vi "ZCAN_Send_Multiframe.vi"(4 "CAN_CH":u8, 5 "CANFD_SpeedUp":u32, 6 "SendData":string="11 22 33 44 55 66 77 88", 7 "ID":u32=18 format="0x%08x", 8 "error in":errorcluster, 9 "agreement":T1, 10 "frame type":T2, 11 "can_index_handle":u32) -> (0 "error out":errorcluster, 3 "Send,DataOut":string)   [LabVIEW 2020]
uses:
  data_type/frame type.ctl
  data_type/Agreement.ctl
  data_type/ZCAN_TransmitFD_frame.ctl
  c76635de-1d19-4bb1-8ca9-fd1db6ddedf1.vi
  zlgcan.lvlib
panel:
  in  "Wait_ms":i32
  in  "Send FillUp":string="AA"
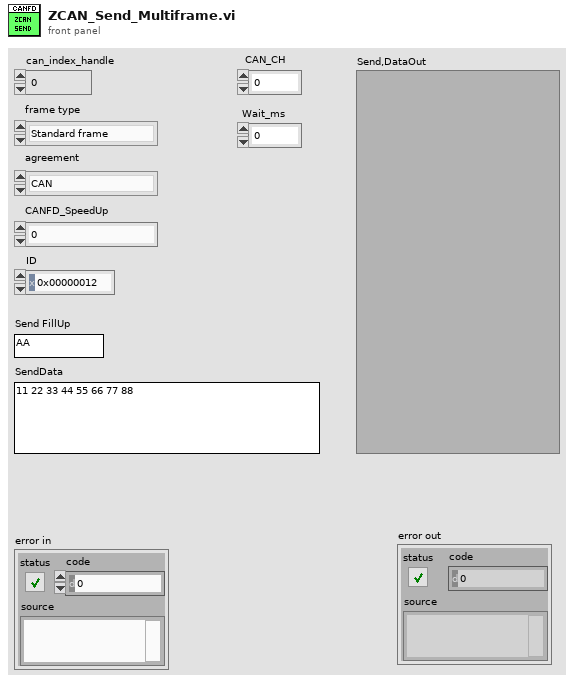
[diagram p1: front panel]
types:
  T1 = typedef "zlgcan.lvlib/Agreement.ctl" = enum16{"CAN", "CANFD"}
  T2 = typedef "zlgcan.lvlib/frame type.ctl" = enum32{"Standard frame", "Extended frame"}
  T3 = typedef "zlgcan.lvlib/ZCAN_TransmitFD_frame.ctl" = cluster{"帧类型":u32, "帧格式":u32, "ID":u32, "数据长度":u8, "CANFD加速？":u8, "DATA":cluster{"CAN数据[0]":u8, "CAN数据[1]":u8, "CAN数据[2]":u8, "CAN数据[3]":u8, "CAN数据[4]":u8, "CAN数据[5]":u8, "CAN数据[6]":u8, "CAN数据[7]":u8, "CAN数据[8]":u8, "CAN数据[9]":u8, "CAN数据[10]":u8, "CAN数据[11] ":u8, "CAN数据[12] ":u8, "CAN数据[13] ":u8, "CAN数据[14] ":u8, "CAN数据[15] ":u8, "CAN数据[16]":u8, "CAN数据[17]":u8, "CAN数据[18]":u8, "CAN数据[19]":u8, "CAN数据[20]":u8, "CAN数据[21]":u8, "CAN数据[22]":u8, "CAN数据[23]":u8, "CAN数据[24] ":u8, "CAN数据[25]":u8, "CAN数据[26]":u8, "CAN数据[27]":u8, "CAN数据[28]":u8, "CAN数据[29]":u8, "CAN数据[30]":u8, "CAN数据[31]":u8, "CAN数据[32]":u8, "CAN数据[33]":u8, "CAN数据[34]":u8, "CAN数据[35]":u8, "CAN数据[36]":u8, "CAN数据[37]":u8, "CAN数据[38]":u8, "CAN数据[39]":u8, "CAN数据[40]":u8, "CAN数据[41]":u8, "CAN数据[42]":u8, "CAN数据[43]":u8, "CAN数据[44]":u8, "CAN数据[45]":u8, "CAN数据[46]":u8, "CAN数据[47]":u8, "CAN数据[48]":u8, "CAN数据[49]":u8, "CAN数据[50]":u8, "CAN数据[51]":u8, "CAN数据[52]":u8, "CAN数据[53]":u8, "CAN数据[54]":u8, "CAN数据[55]":u8, "CAN数据[56]":u8, "CAN数据[57]":u8, "CAN数据[58]":u8, "CAN数据[59]":u8, "CAN数据[60]":u8, "CAN数据[61]":u8, "CAN数据[62]":u8, "CAN数据[63]":u8}}
  T4 = cluster{"u8 Data[][0]":u8, "u8 Data[][1]":u8, "u8 Data[][2]":u8, "u8 Data[][3]":u8, "u8 Data[][4]":u8, "u8 Data[][5]":u8, "u8 Data[][6]":u8, "u8 Data[][7]":u8, "u8 Data[][8]":u8, "u8 Data[][9]":u8, "u8 Data[][10]":u8, "u8 Data[][11]":u8, "u8 Data[][12]":u8, "u8 Data[][13]":u8, "u8 Data[][14]":u8, "u8 Data[][15]":u8, "u8 Data[][16]":u8, "u8 Data[][17]":u8, "u8 Data[][18]":u8, "u8 Data[][19]":u8, "u8 Data[][20]":u8, "u8 Data[][21]":u8, "u8 Data[][22]":u8, "u8 Data[][23]":u8, "u8 Data[][24]":u8, "u8 Data[][25]":u8, "u8 Data[][26]":u8, "u8 Data[][27]":u8, "u8 Data[][28]":u8, "u8 Data[][29]":u8, "u8 Data[][30]":u8, "u8 Data[][31]":u8, "u8 Data[][32]":u8, "u8 Data[][33]":u8, "u8 Data[][34]":u8, "u8 Data[][35]":u8, "u8 Data[][36]":u8, "u8 Data[][37]":u8, "u8 Data[][38]":u8, "u8 Data[][39]":u8, "u8 Data[][40]":u8, "u8 Data[][41]":u8, "u8 Data[][42]":u8, "u8 Data[][43]":u8, "u8 Data[][44]":u8, "u8 Data[][45]":u8, "u8 Data[][46]":u8, "u8 Data[][47]":u8, "u8 Data[][48]":u8, "u8 Data[][49]":u8, "u8 Data[][50]":u8, "u8 Data[][51]":u8, "u8 Data[][52]":u8, "u8 Data[][53]":u8, "u8 Data[][54]":u8, "u8 Data[][55]":u8, "u8 Data[][56]":u8, "u8 Data[][57]":u8, "u8 Data[][58]":u8, "u8 Data[][59]":u8, "u8 Data[][60]":u8, "u8 Data[][61]":u8, "u8 Data[][62]":u8, "u8 Data[][63]":u8}
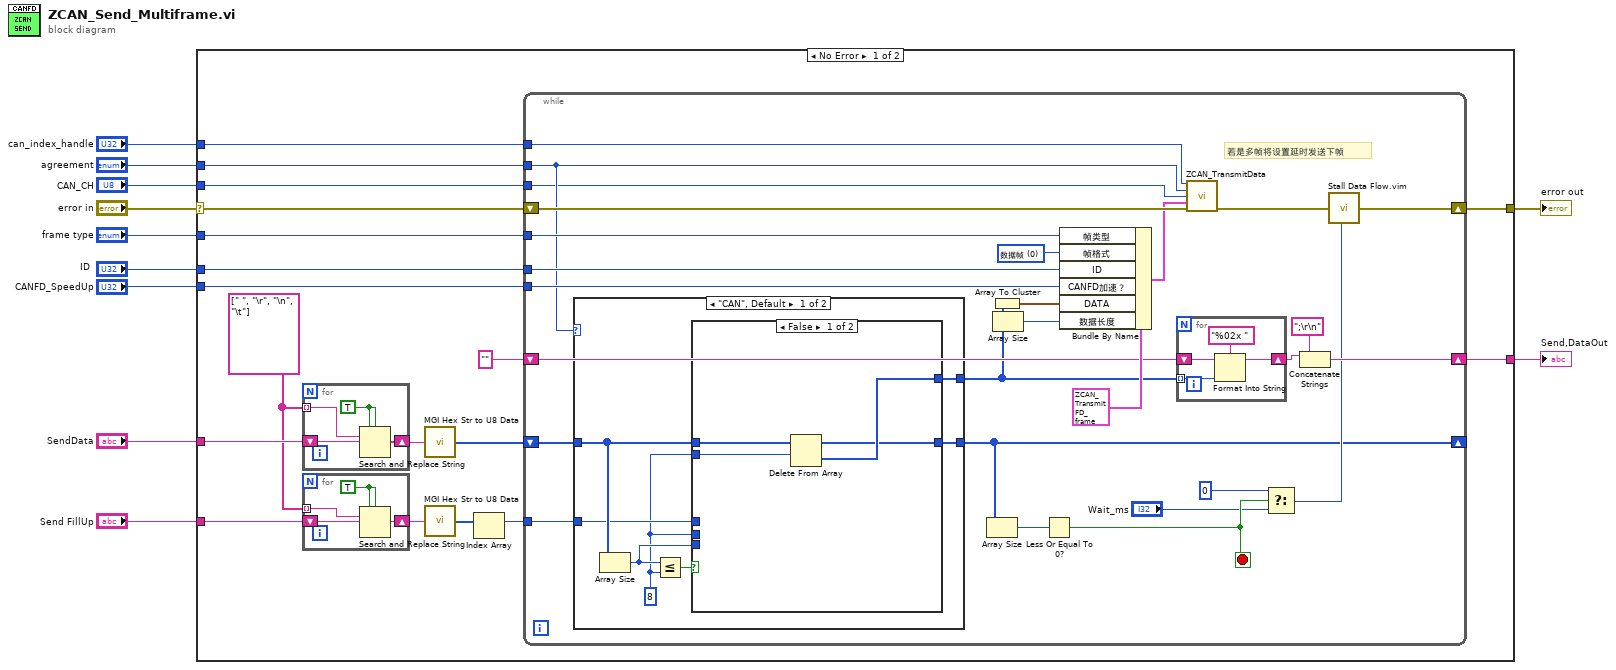
[diagram p0: block diagram]
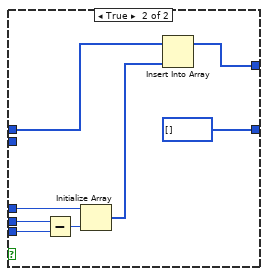
[diagram p2: hidden frame]
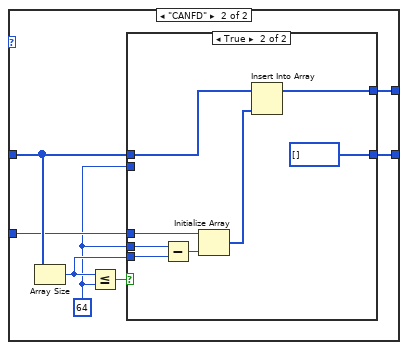
[diagram p3: hidden frame]
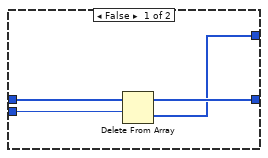
[diagram p4: hidden frame]
diagram:
  n1 = case shown="No Error" "error in" {
    selector: "error in" -> [w29 w108]
    tunnel: [w28 w108] -> w10
    tunnel: "can_index_handle" -> [w27 _]
    tunnel: "frame type" -> [w26 _]
    tunnel: "ID" -> [w25 _]
    tunnel: "CANFD_SpeedUp" -> [w24 _]
    tunnel: "SendData" -> [w22 w107]
    tunnel: "agreement" -> [w18 _]
    tunnel: [w16 w107] -> w3
    tunnel: "CAN_CH" -> [w15 _]
    tunnel: "Send FillUp" -> [w13 _]
    frame No Error {
      w12 = string[] [" ", "\r", "\n", "\t"] ("search string")
      n2 = for {
        tunnel: w12 -> [w35] mode=indexing
        shift-right: [w37] -> w23
        shift-left: w22 -> [w36]
        w34 = TRUE ("replace all? (F)")
        n3 = Search and Replace String(replace all?=w34, case sensitive?=w34, input string=w36, search string=w35) -> (result string=w37:string)  [unwired: 4 in, 3 out]
      }
      n4 = for {
        tunnel: w12 -> [w31] mode=indexing
        shift-right: [w33] -> w14
        shift-left: w13 -> [w32]
        w30 = TRUE ("replace all? (F)")
        n5 = Search and Replace String(replace all?=w30, case sensitive?=w30, input string=w32, search string=w31) -> (result string=w33:string)  [unwired: 4 in, 3 out]
      }
      n6 = call <userlib>:"MGI Hex Str to U8 Data.vi"("HEX String (0-9,A-F)"=w23) -> ("u8 Data[]"=w21:u8[])
      n7 = call <userlib>:"MGI Hex Str to U8 Data.vi"("HEX String (0-9,A-F)"=w14) -> ("u8 Data[]"=w20:u8[])
      n8 = Index Array(array=w20) -> (element=w19:u8)  [unwired: 1 in]
      n9 = while {
        tunnel: w27 -> [w63]
        tunnel: w26 -> [w60]
        tunnel: w25 -> [w58]
        tunnel: w24 -> [w57]
        tunnel: w19 -> [w54]
        tunnel: w18 -> [w53]
        shift-right: [w38] -> w28
        shift-left: w29 -> [w64]
        shift-right: [w40] -> _
        shift-left: w21 -> [w56]
        shift-right: [w47] -> w16
        shift-left: "" -> [w49]
        tunnel: w15 -> [w45]
        stop <- w42 stop-if-true
        w59 = u32 0 items=["数据帧", "远程帧"] ("帧格式")
        # "若是多帧将设置延时发送下帧"
        n10 = case shown="\"CAN\", Default" w53 {
          tunnel: w56 -> [w74 w93]
          tunnel: [w71 w90] -> w48
          tunnel: w54 -> [w72 w91]
          tunnel: [w70 w89] -> w40
          frame "CAN", Default {
            w69 = 8 ("y")
            n11 = Array Size(array=w74) -> (size(s)=w73:i32)
            n12 = Less Or Equal?(x=w73, y=w69) -> (x <= y?=w75:bool)
            n13 = case shown="False" w75 {
              tunnel: w74 -> [w79 w83]
              tunnel: w73 -> [_ w87]
              tunnel: w69 -> [_ w86]
              tunnel: w72 -> [_ w84]
              tunnel: [w77 w81] -> w71
              tunnel: [w76 u8[] [] ("u8 Data[]")] -> w70
              tunnel: w69 -> [w78 _]
              frame False {
                n14 = Delete From Array(array=w79, length=w78) -> (deleted portion=w77:u8[], array with subset deleted=w76:u8[])  [unwired: 1 in]
              }
              frame True {
                n15 = Subtract(x=w86, y=w87) -> (x-y=w85:i32)
                n16 = Initialize Array(w84, w85) -> (w82:u8[])
                n17 = Insert Into Array(array=w83, new element=w82) -> (w81:u8[])  [unwired: 1 in]
              }
            }
          }
          frame "CANFD" {
            w88 = 64 ("y")
            n18 = Array Size(array=w93) -> (size(s)=w92:i32)
            n19 = Less Or Equal?(x=w92, y=w88) -> (x <= y?=w94:bool)
            n20 = case shown="True" w94 {
              tunnel: w93 -> [w98 w102]
              tunnel: w92 -> [_ w106]
              tunnel: w88 -> [_ w105]
              tunnel: w91 -> [_ w103]
              tunnel: [w95 w100] -> w90
              tunnel: [w96 u8[] [] ("u8 Data[]")] -> w89
              tunnel: w88 -> [w97 _]
              frame False {
                n21 = Delete From Array(array=w98, length=w97) -> (deleted portion=w95:u8[], array with subset deleted=w96:u8[])  [unwired: 1 in]
              }
              frame True {
                n22 = Subtract(x=w105, y=w106) -> (x-y=w104:i32)
                n23 = Initialize Array(w103, w104) -> (w101:u8[])
                n24 = Insert Into Array(array=w102, new element=w101) -> (w100:u8[])  [unwired: 1 in]
              }
            }
          }
        }
        n25 = Array Size(array=w40) -> (size(s)=w51:i32)
        n26 = Array To Cluster(array=w48) -> (cluster=w55:T4)
        n27 = Array Size(array=w48) -> (size(s)=w52:i32)
        n28 = Less Or Equal To 0?(x=w51) -> (x <= 0?=w42:bool)
        n29 = Bundle By Name(cluster=T3 {"帧类型"=0, "帧格式"=0, "ID"=0, "数据长度"=0, "CANFD加速？"=0, "DATA"={"CAN数据[0]"=0, "CAN数据[1]"=0, "CAN数据[2]"=0, "CAN数据[3]"=0, "CAN数据[4]"=0, "CAN数据[5]"=0, "CAN数据[6]"=0, "CAN数据[7]"=0, "CAN数据[8]"=0, "CAN数据[9]"=0, "CAN数据[10]"=0, "CAN数据[11] "=0, "CAN数据[12] "=0, "CAN数据[13] "=0, "CAN数据[14] "=0, "CAN数据[15] "=0, "CAN数据[16]"=0, "CAN数据[17]"=0, "CAN数据[18]"=0, "CAN数据[19]"=0, "CAN数据[20]"=0, "CAN数据[21]"=0, "CAN数据[22]"=0, "CAN数据[23]"=0, "CAN数据[24] "=0, "CAN数据[25]"=0, "CAN数据[26]"=0, "CAN数据[27]"=0, "CAN数据[28]"=0, "CAN数据[29]"=0, "CAN数据[30]"=0, "CAN数据[31]"=0, "CAN数据[32]"=0, "CAN数据[33]"=0, "CAN数据[34]"=0, "CAN数据[35]"=0, "CAN数据[36]"=0, "CAN数据[37]"=0, "CAN数据[38]"=0, "CAN数据[39]"=0, "CAN数据[40]"=0, "CAN数据[41]"=0, "CAN数据[42]"=0, "CAN数据[43]"=0, "CAN数据[44]"=0, "CAN数据[45]"=0, "CAN数据[46]"=0, "CAN数据[47]"=0, "CAN数据[48]"=0, "CAN数据[49]"=0, "CAN数据[50]"=0, "CAN数据[51]"=0, "CAN数据[52]"=0, "CAN数据[53]"=0, "CAN数据[54]"=0, "CAN数据[55]"=0, "CAN数据[56]"=0, "CAN数据[57]"=0, "CAN数据[58]"=0, "CAN数据[59]"=0, "CAN数据[60]"=0, "CAN数据[61]"=0, "CAN数据[62]"=0, "CAN数据[63]"=0}} ("canfd_frame"), "帧类型"=w60, "帧格式"=w59, "ID"=w58, "CANFD加速？"=w57, "DATA"=w55, "数据长度"=w52) -> (w61:T3)
        n30 = for {
          shift-right: [w68] -> w50
          shift-left: w49 -> [w67]
          tunnel: w48 -> [w65] mode=indexing
          n31 = Format Into String(format string="%02x ", initial string=w67, w65) -> (resulting string=w68:string)  [unwired: 1 in, 1 out]
        }
        n32 = call "ZCAN_TransmitData.vi"("can_index_handle"=w63, "帧类型"=w53, "CAN通道号"=w45, "canfd_frame"=w61, "error in (no error)"=w64) -> ("error out"=w39:errorcluster)  [unwired: 10 in]
        n33 = Select(t=0, s=w42, f="Wait_ms") -> (s? t:f=w44:i32)
        n34 = Concatenate Strings(w50, ";\r\n" ("string")) -> (w47:string)
        n35 = call "Stall Data Flow.vim"("value in"=w39, "milliseconds to wait"=w44) -> ("value out"=w38:errorcluster)  [unwired: 1 out]
      }
    }
    frame Error {
    }
  }
  "error out" <- w10
  "Send,DataOut" <- w3
